vi "HEWH Adjust Temp.vi"(0 "Core HEWH Data Input":T12={"Scan Rate Adjust"=0.0, "Draw Count"=0, "Test Patten Setup"={"Total Gallons Schedule"=[], "PRAT/RLT Sequence"=[{"Sequence #"=1.0, "Cycles"=35, "Mode Setting"="", "Flow Rate (GPM)"=0.0, "Temperature (F)"=0.0, "Reset Timer"=FALSE, "Use Temp Decline Method"=FALSE, "Terminate Condition"=enum."C1-Terminate Draw @ Gallon Mark", "Condition Value #1"=0.0, "UE"=FALSE, "LE"=FALSE, "Comp"=FALSE, "Fan"=FALSE, "Test End Time (Sec)"=0.0, "Purge Until Cutout"=FALSE, "Start Conditions"=enum."Heat Source Cutout", "Condition Value #2"=0.0, "Remove Power"=FALSE, "Time"=0.0, "Check Special Cond."=enum."SC1-Do Nothing", "Condition#"=enum."C1", "Draw Flags"=enum."N/A", "Data Processing Delay (FHD 15sec, UEF 5 Sec)"=0.0, "Test Complete"=FALSE, "User Setpoint"=0.0, "Tank Setpoint"=0.0}, {"Sequence #"=2.0, "Cycles"=15, "Mode Setting"="", "Flow Rate (GPM)"=0.0, "Temperature (F)"=0.0, "Reset Timer"=FALSE, "Use Temp Decline Method"=FALSE, "Terminate Condition"=enum."C1-Terminate Draw @ Gallon Mark", "Condition Value #1"=0.0, "UE"=FALSE, "LE"=FALSE, "Comp"=FALSE, "Fan"=FALSE, "Test End Time (Sec)"=0.0, "Purge Until Cutout"=FALSE, "Start Conditions"=enum."Heat Source Cutout", "Condition Value #2"=0.0, "Remove Power"=FALSE, "Time"=0.0, "Check Special Cond."=enum."SC1-Do Nothing", "Condition#"=enum."C1", "Draw Flags"=enum."N/A", "Data Processing Delay (FHD 15sec, UEF 5 Sec)"=0.0, "Test Complete"=FALSE, "User Setpoint"=0.0, "Tank Setpoint"=0.0}, {"Sequence #"=3.0, "Cycles"=35, "Mode Setting"="", "Flow Rate (GPM)"=0.0, "Temperature (F)"=0.0, "Reset Timer"=FALSE, "Use Temp Decline Method"=FALSE, "Terminate Condition"=enum."C1-Terminate Draw @ Gallon Mark", "Condition Value #1"=0.0, "UE"=FALSE, "LE"=FALSE, "Comp"=FALSE, "Fan"=FALSE, "Test End Time (Sec)"=0.0, "Purge Until Cutout"=FALSE, "Start Conditions"=enum."Heat Source Cutout", "Condition Value #2"=0.0, "Remove Power"=FALSE, "Time"=0.0, "Check Special Cond."=enum."SC1-Do Nothing", "Condition#"=enum."C1", "Draw Flags"=enum."N/A", "Data Processing Delay (FHD 15sec, UEF 5 Sec)"=0.0, "Test Complete"=FALSE, "User Setpoint"=0.0, "Tank Setpoint"=0.0}, {"Sequence #"=4.0, "Cycles"=15, "Mode Setting"="", "Flow Rate (GPM)"=0.0, "Temperature (F)"=0.0, "Reset Timer"=FALSE, "Use Temp Decline Method"=FALSE, "Terminate Condition"=enum."C1-Terminate Draw @ Gallon Mark", "Condition Value #1"=0.0, "UE"=FALSE, "LE"=FALSE, "Comp"=FALSE, "Fan"=FALSE, "Test End Time (Sec)"=0.0, "Purge Until Cutout"=FALSE, "Start Conditions"=enum."Heat Source Cutout", "Condition Value #2"=0.0, "Remove Power"=FALSE, "Time"=0.0, "Check Special Cond."=enum."SC1-Do Nothing", "Condition#"=enum."C1", "Draw Flags"=enum."N/A", "Data Processing Delay (FHD 15sec, UEF 5 Sec)"=0.0, "Test Complete"=FALSE, "User Setpoint"=0.0, "Tank Setpoint"=0.0}, {"Sequence #"=5.0, "Cycles"=35, "Mode Setting"="", "Flow Rate (GPM)"=0.0, "Temperature (F)"=0.0, "Reset Timer"=FALSE, "Use Temp Decline Method"=FALSE, "Terminate Condition"=enum."C1-Terminate Draw @ Gallon Mark", "Condition Value #1"=0.0, "UE"=FALSE, "LE"=FALSE, "Comp"=FALSE, "Fan"=FALSE, "Test End Time (Sec)"=0.0, "Purge Until Cutout"=FALSE, "Start Conditions"=enum."Heat Source Cutout", "Condition Value #2"=0.0, "Remove Power"=FALSE, "Time"=0.0, "Check Special Cond."=enum."SC1-Do Nothing", "Condition#"=enum."C1", "Draw Flags"=enum."N/A", "Data Processing Delay (FHD 15sec, UEF 5 Sec)"=0.0, "Test Complete"=FALSE, "User Setpoint"=0.0, "Tank Setpoint"=0.0}, {"Sequence #"=6.0, "Cycles"=15, "Mode Setting"="", "Flow Rate (GPM)"=0.0, "Temperature (F)"=0.0, "Reset Timer"=FALSE, "Use Temp Decline Method"=FALSE, "Terminate Condition"=enum."C1-Terminate Draw @ Gallon Mark", "Condition Value #1"=0.0, "UE"=FALSE, "LE"=FALSE, "Comp"=FALSE, "Fan"=FALSE, "Test End Time (Sec)"=0.0, "Purge Until Cutout"=FALSE, "Start Conditions"=enum."Heat Source Cutout", "Condition Value #2"=0.0, "Remove Power"=FALSE, "Time"=0.0, "Check Special Cond."=enum."SC1-Do Nothing", "Condition#"=enum."C1", "Draw Flags"=enum."N/A", "Data Processing Delay (FHD 15sec, UEF 5 Sec)"=0.0, "Test Complete"=FALSE, "User Setpoint"=0.0, "Tank Setpoint"=0.0}, {"Sequence #"=7.0, "Cycles"=35, "Mode Setting"="", "Flow Rate (GPM)"=0.0, "Temperature (F)"=0.0, "Reset Timer"=FALSE, "Use Temp Decline Method"=FALSE, "Terminate Condition"=enum."C1-Terminate Draw @ Gallon Mark", "Condition Value #1"=0.0, "UE"=FALSE, "LE"=FALSE, "Comp"=FALSE, "Fan"=FALSE, "Test End Time (Sec)"=0.0, "Purge Until Cutout"=FALSE, "Start Conditions"=enum."Heat Source Cutout", "Condition Value #2"=0.0, "Remove Power"=FALSE, "Time"=0.0, "Check Special Cond."=enum."SC1-Do Nothing", "Condition#"=enum."C1", "Draw Flags"=enum."N/A", "Data Processing Delay (FHD 15sec, UEF 5 Sec)"=0.0, "Test Complete"=FALSE, "User Setpoint"=0.0, "Tank Setpoint"=0.0}, {"Sequence #"=8.0, "Cycles"=15, "Mode Setting"="", "Flow Rate (GPM)"=0.0, "Temperature (F)"=0.0, "Reset Timer"=FALSE, "Use Temp Decline Method"=FALSE, "Terminate Condition"=enum."C1-Terminate Draw @ Gallon Mark", "Condition Value #1"=0.0, "UE"=FALSE, "LE"=FALSE, "Comp"=FALSE, "Fan"=FALSE, "Test End Time (Sec)"=0.0, "Purge Until Cutout"=FALSE, "Start Conditions"=enum."Heat Source Cutout", "Condition Value #2"=0.0, "Remove Power"=FALSE, "Time"=0.0, "Check Special Cond."=enum."SC1-Do Nothing", "Condition#"=enum."C1", "Draw Flags"=enum."N/A", "Data Processing Delay (FHD 15sec, UEF 5 Sec)"=0.0, "Test Complete"=FALSE, "User Setpoint"=0.0, "Tank Setpoint"=0.0}], "Current Sequence Index"=0}, "HEWH Specific DAQ"={"HEWH Data"={"HEWH Standard"={"Voltage (Volts)"=0.0, "Current (Amps)"=0.0, "Power (Watts)"=0.0, "WattHours (Wh)"=0.0, "TC Tree (AVG)"=0.0, "Flow Rate (GPM)"=0.0, "Gallons (Gal)"=0.0, "RTD Out (Deg F)"=0.0, "RTD In (Deg F)"=0.0, "RTD Amb (Deg F)"=0.0, "TC Down"=0.0, "UE Event Lead"=0, "LE Event Lead"=0, "TC 8"=0.0, "TC 9"=0.0, "TC 10"=0.0, "TC Tree Array (1-6)"=[], "TC 7"=0.0, "PSI 1"=0.0, "PSI 2"=0.0, "PSI 3"=0.0, "PSI 4"=0.0, "Gas BTU"=0.0, "Gas BTU/hr"=0.0}, "PRAT"={"Power (Watts) A"=4192.0, "Power (Watts) B"=4192.0, "Power (Watts) C"=4192.0, "Power (Watts) D"=4192.0, "TC1"=0.0, "TC2"=0.0, "TC3"=0.0, "TC4"=0.0, "WattHours (Wh) A"=4192.0, "WattHours (Wh) B"=4192.0, "WattHours (Wh) C"=4192.0, "WattHours (Wh) D"=4192.0, "Ambient"=0.0, "Extra Temp"=0.0}, "Additional Power Data"={"Vthd"=236.2, "Frequency (Hz)"=236.2, "Apparent Power (VA)"=236.2, "Power Factor"=236.2, "Current Crest Factor"=236.2, "Voltage Crest Factor"=236.2, "Integration Time (sec)"=236.2}}, "Flow Valve % Open"=0.0, "Power State"={"UE"=FALSE, "LE"=FALSE, "COMP"=FALSE, "FANS"=FALSE}, "Power Analyzer"=enum."APLUS", "Flow Valve uA Output"=0, "Gallons Start (Gal)"=0.0, "PI Output"=0.0}, "Test Output Data"={"PreDraw Data Table"=[], "Data Table"=[], "MW100 TC Headers"=[]}, "Calc and Calibration"={"Mean SD Var Max Min Array"=[], "Draw Statistics (DBL)"=[], "Calibration Coefficients DBL"=[], "Start Gallons"=0.0, "Starting Temp Decline"=0.0, "K-Factor (Temperature)"=0.0, "All Draw Stats"=[], "RTD Terminate Value"=0.0, "K-Factor (Flow)"=0.0, "Intellifaucet Type"="", "Thermal Stabil Array"=[], "Gas Thermal Stabil Complete"=FALSE, "Therm Reset Cmpt 1"=FALSE, "Therm Reset Cmpt 2"=FALSE, "Last Flow Rate (Therm)"=0.0, "State"=enum."State 1", "Gas Thermal Time"=0.0, "Target Rate (Thermal)"=0.0, "Thermal - Final"=[], "State5 Gal Water"=0.0, "State 5 Gal Gas"=0.0, "Intellif Open < 1"=0.0, "Intellif Open < 1.7"=0.0, "Intellif Open < 2.2"=0.0, "Intellif Open > 2.2"=0.0, "End of Draw\nComparison"=[]}, "Current Draw Time"=0.0, "LV Program"=enum."HEWH", "Station ID"=enum."A", "Current Cond"=enum."N/A", "Test Complete"=FALSE, "ANSI Rate"={"Array 1"=[], "Array 3"=[], "Array 2"=[], "Start ANSI"=FALSE, "ANSI Start Time"=0.0, "Restart ANSI"=FALSE, "15 Min ANSI Avg (BTU/hr)"=0.0, "20 Min ANSI Avg (BTU/hr)"=0.0, "25 Min ANSI Avg (BTU/hr)"=0.0, "Absolute Pressure"=0.0, "Gas Temperature"=0.0, "Volumetric Flow Rate"=0.0, "Mass Flow Rate"=0.0, "Array 4"=[], "Array 5"=[], "Gas Rate"=0.0, "15 Min Pres Avg (PSIA)"=0.0, "20 Min Pres Avg (PSIA)"=0.0, "25 Min Pres Avg (PSIA)"=0.0, "15 Min Temp Avg (°F) "=0.0, "20 Min Temp Avg (°F)"=0.0, "25 Min Temp Avg (°F)"=0.0, "15 Min Uncorrected Avg (CFH)"=0.0, "20 Min Uncorrected Avg (CFH)"=0.0, "25 Min Uncorrected Avg (CFH)"=0.0, "15 Min Corrected Avg (SCFH)"=0.0, "20 Min Corrected Avg (SCFH)"=0.0, "25 Min Corrected Avg (SCFH)"=0.0, "15 Min Complete"=FALSE, "20 Min Complete"=FALSE, "25 Min Complete"=FALSE, "Heating Value (BTU/ft³)"=0.0, "CO CO2 15 Min"=[], "CO CO2 20 Min"=[], "CO CO2 25 Min"=[], "CO CO2 Real Time"=[]}, "Module 4 Relay Status"={"INTELLIFAUCET TEMP(T)/FLOW(F) (CH 041)"=FALSE, "INTELLIFAUCET READY (CH 042)"=FALSE, "INTELLIFAUCET START (CH 043)"=FALSE, "INTELLIFAUCET STOP (CH 044)"=FALSE, "MAIN POWER RELAY (CH 047)"=FALSE, "NOT USED (CH 045)"=FALSE, "NOT USED (CH 046)"=FALSE, "PURGE VALVE RELAY (CH 048)"=FALSE, "OUTLET VALVE RELAY (CH 049)"=FALSE, "INLET VALVE RELAY (CH 050)"=FALSE, "Intellifaucet (% Open)"=0.0, "Proportioning Valve (%Open)"=0.0, "Intellifaucet Temp Setpoint (F)"=0.0}, "Inficon Data Output"={"Gross Heating Value, Vol (Real, Dry)"=1067.4462890625, "Nitrogen Component Normalized Mole % (Dry)"=0.0, "Methane Component Normalized Mole % (Dry)"=92.87550354003906, "Carbon Dioxide Component Normalized Mole % (Dry)"=0.1941000074148178, "Ethane Component Normalized Mole % (Dry)"=6.454999923706055, "Propane Component Normalized Mole % (Dry)"=0.3865000009536743, "i-Pentane Component Normalized Mole % (Dry)"=0.007799999788403511, "i-Butane Component Normalized Mole % (Dry)"=0.03880000114440918, "n-Butane Component Normalized Mole % (Dry)"=0.03819999843835831, "n-Pentane Component Normalized Mole % (Dry)"=0.004100000020116568, "Hexane Component Normalized Mole % (Dry)"=0.0, "Heptane Component Normalized Mole % (Dry)"=0.0, "Gross Wobbe Index, Real(Dry)"=1385.8905029296875, "Relative Density, Real(Dry)"=0.5932452082633972, "Propylene Component Normalized Mole % (Dry)"=0.0, "C4 Olefins Component Normalized Mole % (Dry)"=0.0, "Water Component Normalized Mole % (Dry)"=0.0, "Gross Heating Value, Vol (Real, Sat)"=0.0}, "Gas Measurements"={"Gas Measurment Data -Alicat"={"Absolute Pressure"=0.0, "Gauge/Diff. Pressure"=0.0, "Barometric Pressure"=0.0, "Temperature"=0.0, "Volumetric Flow"=0.0, "Mass Flow"=0.0, "Setpoint"=0.0, "Valve Drive"=0.0, "Totalizer"=0.0, "[hr]"=0.0, "[min]"=0.0, "[sec]"=0.0, "Totalizer Average Flow"=0.0, "Totalizer Peak Flow"=0.0, "Gas selected"=""}, "Gas Measurment Data - Ritter"={"Gas Flow Rate (L/hr)-Uncorrected"=0.0, "Totalized Flow (L)--Uncorrected"=0.0, "Gas Flow Rate (cuft/hr)-Uncorrected"=0.0, "Totalized Flow (cuft)-Uncorrected"=0.0, "Gas Temperature (F)"=0.0, "Gas Pressure (in WC)"=0.0, "Heise Barometric Pressure (inHG)"=0.0, "STP Correction Factor"=0.0, "Temp Correction Factor"=0.0, "Pressure Correction Factor"=0.0, "Water Vapor Pressure"=0.0, "Gas Flow Rate (cuft/hr)-Corrected"=0.0, "Totalized Flow (cuft)-Corrected"=0.0}}} {"Test Patten Setup"."PRAT/RLT Sequence"."Time" format="%<%H:%M:%S>t"; "Test Patten Setup"."Total Gallons Schedule" format="%.2f"}, 1 "Test Fixture Hardware":T1={"Power "={"Yokogawa"={"WT210"={"Sample Rate (1: 0.25s)"=1, "A Range (12: 20A)"=11, "V Range (6: 600V)"=4, "Power VISA Yokogawa WT210"="WT210"}, "WT500"={"Power VISA Yokogawa WT500"="", "V Range (8: 1000V)"=6, "I Range (7: 40A)"=7, "Update Rate (3: 500ms)"=2}, "WT310_2"={"Sample Rate (1: 0.25s)"=1, "A Range (12: 20A)"=11, "V Range (6: 600V)"=4, "Power VISA Yokogawa WT310_2"="WT310_2"}, "WT310_3"={"Sample Rate (1: 0.25s)"=1, "A Range (12: 20A)"=11, "V Range (6: 600V)"=4, "Power VISA Yokogawa WT310_3"="WT310_3"}}, "Aplus"={"Aplus IP Address"="192.168.1.101", "Remote Port"=502, "Instrument"="APLUS", "Instr Driver Revision"="1.03.0053"}, "Power Limits"={"Crest Factor"={"Upper Limit"=1.49, "Lower Limit"=1.34}, "Harmonic Content"={"Uthd"=2.0}, "Voltage"={"% Error"=2.0}, "Stability"={"<1 Watt "={"Wattage"=1.0, "Slope (mW/H)"=10.0}, ">1 Watt"={"1%Power/Hour"=1.0}}}, "Nominal Voltage"=120, "Time Limit (s)"=10800.0, "Power Variation Limit (%)"=50.0, "Power Supply"={"Chroma 61605"="CHROMA", "Use Chroma?"=FALSE}}, "Weight Scale"={"Com Options"={"IND560Scale VISA"="IND560", "IP Address"="", "Remote Port"=502, "Setra Scale VISA"="SETRA", "GSE 350"="GSE350"}, "Select Scale"=""}, "Flow Rates"={"Laurel Cold IP Address"="", "Laurel Hot IP Address"="", "Hot Water Laurel VISA"="LaurelMeter_Hot", "Cold Water Laurel VISA"="LaurelMeter_Cold", "Remote Port"=0, "Laurel Communication Type"="", "Meters To Collect (Hot Cold)"="", "HOT Laurel Reference"=refnum, "COLD Laurel Reference"=refnum, "Modbus Hot Ref"=refnum}, "Analog Data"={"Agilent"={"Agilent 34972_1"="34972A_1", "Agilent 34972_2"="34972A_2", "Agilent 34972_3"="34972A_3", "Agilent 34972_4"="34972A_3", "Agilent 34972_5"="34972A_3", "Agilent 34972_6"="34972A_3", "Agilent Gain"=0.0, "TC Type (K,J,T)"="", "Instrument IDN?"="", "TC Channels-List"="", "Analog Channels-List"="", "Agilent Cluster Array"=[], "TC Channels-List 2"="", "Analog Channels-List 2"=""}, "Yokogawa"={"MW100"="MW100", "Intellifaucet"=FALSE}, "Select Analog"="", "TC Coefficients"={"TC Coefficients 1"=[], "TC Coefficients 2"=[], "TC Coefficients 3"=[], "TC Coefficients 4"=[], "TC Coefficients 5"=[], "TC Coefficients 6"=[], "TC Coefficients 7"=[]}, "NI Tasks (Dryer DOE)"=["TC Temps-Module 1", "TC Temps-Module 2", "TC Temps-Module 3", "TC Temps-Module 4", "TC Temps-Module 5", "Gas and Temp-Module 6", "AC_DC Events-Module 7"], "Laurel Analog"={"Laurel IP (Water Temp)"="", "Laurel IP (Pressure)"=""}}, "ITHX-Temp Humidity"={"IP Address 1"="", "Remote Port"=0, "IP Address 2"="", "IP Address 3"=""}, "Gas Meter"={"Gas Meter 1"="COM3", "Gas Meter 2"="COM4", "Gas Meter 3"="COM5", "Gas Meter 4"="COM6", "Gas Meter 5"="COM7", "Gas Meter 6"="COM8", "Data Frame Format"={"Absolute Pressure"=FALSE, "Gauge/Diff. Pressure"=FALSE, "Barometric Pressure"=FALSE, "Temperature"=FALSE, "Volumetric"=FALSE, "Mass"=FALSE, "Setpoint"=FALSE, "Valve Drive"=FALSE, "Totalizer"=FALSE, "Totalizer Timer"=FALSE, "Totalizer Average Flow"=FALSE, "Totalizer Peak Flow"=FALSE, "Gas Selected"=FALSE, "Tot. Timer Format"=0}, "Measurement Units"={"Software Rev"="", "Model Number"="", "Manufacturer Info"="", "Software Sub-Rev"="", "Board Rev"="", "Units of Measure Input"={"Abs. Pressure"="", "Gauge/Diff. Press."="", "Barometric Press."="", "Temperature"="", "Volume"="", "Mass"="", "Setpoint"="", "Valve Drive"="", "Totalizer"="", "Tot. Timer"="", "Tot. Avg. Flow"="", "Tot. Peak Flow"=""}}, "Ritter Gas Meter 1"="COM8"}, "Barometric Pressure"={"HEISE 901A"="HEISE", "Use Barometer?"=FALSE}, "Gas Analysis"={"Ultramat 23 VISA"="ULTRAMAT"}, "Inficon Micro GC"={"Propane IP Address"="192.168.1.33", "Natural Gas  IP Address"="192.168.1.32", "Remote Port"=502, "Natural Modbus"=refnum, "Propane Modbus"=refnum}} {"Power"."Yokogawa"."WT310_3"."V Range (6: 600V)" items=["Auto", "15V", "30V", "60V", "150V", "300V", "600V"]; "Power"."Yokogawa"."WT310_3"."A Range (12: 20A)" items=["Auto", "5mA", "10mA", "20mA", "50mA", "100mA", "200mA", "0.5A", "1A", "2A", "5A", "10A", "20A", "50mV", "100mV", "200mV", "2.5V", "5V", "10V"]; "Power"."Yokogawa"."WT310_3"."Sample Rate (1: 0.25s)" items=["0.1s", "0.25s", "0.5s", "1s", "2s", "5s"]; "Power"."Yokogawa"."WT310_2"."V Range (6: 600V)" items=["Auto", "15V", "30V", "60V", "150V", "300V", "600V"]; "Power"."Yokogawa"."WT310_2"."A Range (12: 20A)" items=["Auto", "5mA", "10mA", "20mA", "50mA", "100mA", "200mA", "0.5A", "1A", "2A", "5A", "10A", "20A", "50mV", "100mV", "200mV", "2.5V", "5V", "10V"]; "Power"."Yokogawa"."WT310_2"."Sample Rate (1: 0.25s)" items=["0.1s", "0.25s", "0.5s", "1s", "2s", "5s"]; "Power"."Yokogawa"."WT500"."Update Rate (3: 500ms)" items=["-", "100ms", "200ms", "500ms", "1s", "2s", "5s"]; "Power"."Yokogawa"."WT500"."I Range (7: 40A)" items=["AUTO", "500 mA", "1 A", "2 A", "5 A", "10 A", "20 A", "40 A", "S-AUTO", "50 mV", "100 mV", "200 mV", "500 mV", "1 V", "2 V", "5 V", "10 V", "250 mA", "500 mA", "1 A", "2.5 A", "5 A", "10 A", "20 A", "25 mV", "50 mV", "100 mV", "250 mV", "500 mV", "1 V", "2.5 V", "5 V"]; "Power"."Yokogawa"."WT500"."V Range (8: 1000V)" items=["AUTO", "15", "30", "60", "100", "150", "300", "600", "1000", "7.5", "15", "30", "50", "75", "150", "300", "500"]; "Power"."Yokogawa"."WT210"."V Range (6: 600V)" items=["Auto", "15V", "30V", "60V", "150V", "300V", "600V"]; "Power"."Yokogawa"."WT210"."A Range (12: 20A)" items=["Auto", "5mA", "10mA", "20mA", "50mA", "100mA", "200mA", "0.5A", "1A", "2A", "5A", "10A", "20A", "50mV", "100mV", "200mV", "2.5V", "5V", "10V"]; "Power"."Yokogawa"."WT210"."Sample Rate (1: 0.25s)" items=["0.1s", "0.25s", "0.5s", "1s", "2s", "5s"]}, 4 "MW100 Sema":T11, 5 "error in (no error)":errorcluster, 7 "Debug":bool, 9 "Temperature":T32 format="%.2f", 13 "Adjust Temp":bool) -> (14 "Core HEWH Data Output":T12={"Scan Rate Adjust"=0.0, "Draw Count"=0, "Test Patten Setup"={"Total Gallons Schedule"=[], "PRAT/RLT Sequence"=[{"Sequence #"=1.0, "Cycles"=35, "Mode Setting"="", "Flow Rate (GPM)"=0.0, "Temperature (F)"=0.0, "Reset Timer"=FALSE, "Use Temp Decline Method"=FALSE, "Terminate Condition"=enum."C1-Terminate Draw @ Gallon Mark", "Condition Value #1"=0.0, "UE"=FALSE, "LE"=FALSE, "Comp"=FALSE, "Fan"=FALSE, "Test End Time (Sec)"=0.0, "Purge Until Cutout"=FALSE, "Start Conditions"=enum."Heat Source Cutout", "Condition Value #2"=0.0, "Remove Power"=FALSE, "Time"=0.0, "Check Special Cond."=enum."SC1-Do Nothing", "Condition#"=enum."C1", "Draw Flags"=enum."N/A", "Data Processing Delay (FHD 15sec, UEF 5 Sec)"=0.0, "Test Complete"=FALSE, "User Setpoint"=0.0, "Tank Setpoint"=0.0}, {"Sequence #"=2.0, "Cycles"=15, "Mode Setting"="", "Flow Rate (GPM)"=0.0, "Temperature (F)"=0.0, "Reset Timer"=FALSE, "Use Temp Decline Method"=FALSE, "Terminate Condition"=enum."C1-Terminate Draw @ Gallon Mark", "Condition Value #1"=0.0, "UE"=FALSE, "LE"=FALSE, "Comp"=FALSE, "Fan"=FALSE, "Test End Time (Sec)"=0.0, "Purge Until Cutout"=FALSE, "Start Conditions"=enum."Heat Source Cutout", "Condition Value #2"=0.0, "Remove Power"=FALSE, "Time"=0.0, "Check Special Cond."=enum."SC1-Do Nothing", "Condition#"=enum."C1", "Draw Flags"=enum."N/A", "Data Processing Delay (FHD 15sec, UEF 5 Sec)"=0.0, "Test Complete"=FALSE, "User Setpoint"=0.0, "Tank Setpoint"=0.0}, {"Sequence #"=3.0, "Cycles"=35, "Mode Setting"="", "Flow Rate (GPM)"=0.0, "Temperature (F)"=0.0, "Reset Timer"=FALSE, "Use Temp Decline Method"=FALSE, "Terminate Condition"=enum."C1-Terminate Draw @ Gallon Mark", "Condition Value #1"=0.0, "UE"=FALSE, "LE"=FALSE, "Comp"=FALSE, "Fan"=FALSE, "Test End Time (Sec)"=0.0, "Purge Until Cutout"=FALSE, "Start Conditions"=enum."Heat Source Cutout", "Condition Value #2"=0.0, "Remove Power"=FALSE, "Time"=0.0, "Check Special Cond."=enum."SC1-Do Nothing", "Condition#"=enum."C1", "Draw Flags"=enum."N/A", "Data Processing Delay (FHD 15sec, UEF 5 Sec)"=0.0, "Test Complete"=FALSE, "User Setpoint"=0.0, "Tank Setpoint"=0.0}, {"Sequence #"=4.0, "Cycles"=15, "Mode Setting"="", "Flow Rate (GPM)"=0.0, "Temperature (F)"=0.0, "Reset Timer"=FALSE, "Use Temp Decline Method"=FALSE, "Terminate Condition"=enum."C1-Terminate Draw @ Gallon Mark", "Condition Value #1"=0.0, "UE"=FALSE, "LE"=FALSE, "Comp"=FALSE, "Fan"=FALSE, "Test End Time (Sec)"=0.0, "Purge Until Cutout"=FALSE, "Start Conditions"=enum."Heat Source Cutout", "Condition Value #2"=0.0, "Remove Power"=FALSE, "Time"=0.0, "Check Special Cond."=enum."SC1-Do Nothing", "Condition#"=enum."C1", "Draw Flags"=enum."N/A", "Data Processing Delay (FHD 15sec, UEF 5 Sec)"=0.0, "Test Complete"=FALSE, "User Setpoint"=0.0, "Tank Setpoint"=0.0}, {"Sequence #"=5.0, "Cycles"=35, "Mode Setting"="", "Flow Rate (GPM)"=0.0, "Temperature (F)"=0.0, "Reset Timer"=FALSE, "Use Temp Decline Method"=FALSE, "Terminate Condition"=enum."C1-Terminate Draw @ Gallon Mark", "Condition Value #1"=0.0, "UE"=FALSE, "LE"=FALSE, "Comp"=FALSE, "Fan"=FALSE, "Test End Time (Sec)"=0.0, "Purge Until Cutout"=FALSE, "Start Conditions"=enum."Heat Source Cutout", "Condition Value #2"=0.0, "Remove Power"=FALSE, "Time"=0.0, "Check Special Cond."=enum."SC1-Do Nothing", "Condition#"=enum."C1", "Draw Flags"=enum."N/A", "Data Processing Delay (FHD 15sec, UEF 5 Sec)"=0.0, "Test Complete"=FALSE, "User Setpoint"=0.0, "Tank Setpoint"=0.0}, {"Sequence #"=6.0, "Cycles"=15, "Mode Setting"="", "Flow Rate (GPM)"=0.0, "Temperature (F)"=0.0, "Reset Timer"=FALSE, "Use Temp Decline Method"=FALSE, "Terminate Condition"=enum."C1-Terminate Draw @ Gallon Mark", "Condition Value #1"=0.0, "UE"=FALSE, "LE"=FALSE, "Comp"=FALSE, "Fan"=FALSE, "Test End Time (Sec)"=0.0, "Purge Until Cutout"=FALSE, "Start Conditions"=enum."Heat Source Cutout", "Condition Value #2"=0.0, "Remove Power"=FALSE, "Time"=0.0, "Check Special Cond."=enum."SC1-Do Nothing", "Condition#"=enum."C1", "Draw Flags"=enum."N/A", "Data Processing Delay (FHD 15sec, UEF 5 Sec)"=0.0, "Test Complete"=FALSE, "User Setpoint"=0.0, "Tank Setpoint"=0.0}, {"Sequence #"=7.0, "Cycles"=35, "Mode Setting"="", "Flow Rate (GPM)"=0.0, "Temperature (F)"=0.0, "Reset Timer"=FALSE, "Use Temp Decline Method"=FALSE, "Terminate Condition"=enum."C1-Terminate Draw @ Gallon Mark", "Condition Value #1"=0.0, "UE"=FALSE, "LE"=FALSE, "Comp"=FALSE, "Fan"=FALSE, "Test End Time (Sec)"=0.0, "Purge Until Cutout"=FALSE, "Start Conditions"=enum."Heat Source Cutout", "Condition Value #2"=0.0, "Remove Power"=FALSE, "Time"=0.0, "Check Special Cond."=enum."SC1-Do Nothing", "Condition#"=enum."C1", "Draw Flags"=enum."N/A", "Data Processing Delay (FHD 15sec, UEF 5 Sec)"=0.0, "Test Complete"=FALSE, "User Setpoint"=0.0, "Tank Setpoint"=0.0}, {"Sequence #"=8.0, "Cycles"=15, "Mode Setting"="", "Flow Rate (GPM)"=0.0, "Temperature (F)"=0.0, "Reset Timer"=FALSE, "Use Temp Decline Method"=FALSE, "Terminate Condition"=enum."C1-Terminate Draw @ Gallon Mark", "Condition Value #1"=0.0, "UE"=FALSE, "LE"=FALSE, "Comp"=FALSE, "Fan"=FALSE, "Test End Time (Sec)"=0.0, "Purge Until Cutout"=FALSE, "Start Conditions"=enum."Heat Source Cutout", "Condition Value #2"=0.0, "Remove Power"=FALSE, "Time"=0.0, "Check Special Cond."=enum."SC1-Do Nothing", "Condition#"=enum."C1", "Draw Flags"=enum."N/A", "Data Processing Delay (FHD 15sec, UEF 5 Sec)"=0.0, "Test Complete"=FALSE, "User Setpoint"=0.0, "Tank Setpoint"=0.0}], "Current Sequence Index"=0}, "HEWH Specific DAQ"={"HEWH Data"={"HEWH Standard"={"Voltage (Volts)"=0.0, "Current (Amps)"=0.0, "Power (Watts)"=0.0, "WattHours (Wh)"=0.0, "TC Tree (AVG)"=0.0, "Flow Rate (GPM)"=0.0, "Gallons (Gal)"=0.0, "RTD Out (Deg F)"=0.0, "RTD In (Deg F)"=0.0, "RTD Amb (Deg F)"=0.0, "TC Down"=0.0, "UE Event Lead"=0, "LE Event Lead"=0, "TC 8"=0.0, "TC 9"=0.0, "TC 10"=0.0, "TC Tree Array (1-6)"=[], "TC 7"=0.0, "PSI 1"=0.0, "PSI 2"=0.0, "PSI 3"=0.0, "PSI 4"=0.0, "Gas BTU"=0.0, "Gas BTU/hr"=0.0}, "PRAT"={"Power (Watts) A"=4192.0, "Power (Watts) B"=4192.0, "Power (Watts) C"=4192.0, "Power (Watts) D"=4192.0, "TC1"=0.0, "TC2"=0.0, "TC3"=0.0, "TC4"=0.0, "WattHours (Wh) A"=4192.0, "WattHours (Wh) B"=4192.0, "WattHours (Wh) C"=4192.0, "WattHours (Wh) D"=4192.0, "Ambient"=0.0, "Extra Temp"=0.0}, "Additional Power Data"={"Vthd"=236.2, "Frequency (Hz)"=236.2, "Apparent Power (VA)"=236.2, "Power Factor"=236.2, "Current Crest Factor"=236.2, "Voltage Crest Factor"=236.2, "Integration Time (sec)"=236.2}}, "Flow Valve % Open"=0.0, "Power State"={"UE"=FALSE, "LE"=FALSE, "COMP"=FALSE, "FANS"=FALSE}, "Power Analyzer"=enum."APLUS", "Flow Valve uA Output"=0, "Gallons Start (Gal)"=0.0, "PI Output"=0.0}, "Test Output Data"={"PreDraw Data Table"=[], "Data Table"=[], "MW100 TC Headers"=[]}, "Calc and Calibration"={"Mean SD Var Max Min Array"=[], "Draw Statistics (DBL)"=[], "Calibration Coefficients DBL"=[], "Start Gallons"=0.0, "Starting Temp Decline"=0.0, "K-Factor (Temperature)"=0.0, "All Draw Stats"=[], "RTD Terminate Value"=0.0, "K-Factor (Flow)"=0.0, "Intellifaucet Type"="", "Thermal Stabil Array"=[], "Gas Thermal Stabil Complete"=FALSE, "Therm Reset Cmpt 1"=FALSE, "Therm Reset Cmpt 2"=FALSE, "Last Flow Rate (Therm)"=0.0, "State"=enum."State 1", "Gas Thermal Time"=0.0, "Target Rate (Thermal)"=0.0, "Thermal - Final"=[], "State5 Gal Water"=0.0, "State 5 Gal Gas"=0.0, "Intellif Open < 1"=0.0, "Intellif Open < 1.7"=0.0, "Intellif Open < 2.2"=0.0, "Intellif Open > 2.2"=0.0, "End of Draw\nComparison"=[]}, "Current Draw Time"=0.0, "LV Program"=enum."HEWH", "Station ID"=enum."A", "Current Cond"=enum."N/A", "Test Complete"=FALSE, "ANSI Rate"={"Array 1"=[], "Array 3"=[], "Array 2"=[], "Start ANSI"=FALSE, "ANSI Start Time"=0.0, "Restart ANSI"=FALSE, "15 Min ANSI Avg (BTU/hr)"=0.0, "20 Min ANSI Avg (BTU/hr)"=0.0, "25 Min ANSI Avg (BTU/hr)"=0.0, "Absolute Pressure"=0.0, "Gas Temperature"=0.0, "Volumetric Flow Rate"=0.0, "Mass Flow Rate"=0.0, "Array 4"=[], "Array 5"=[], "Gas Rate"=0.0, "15 Min Pres Avg (PSIA)"=0.0, "20 Min Pres Avg (PSIA)"=0.0, "25 Min Pres Avg (PSIA)"=0.0, "15 Min Temp Avg (°F) "=0.0, "20 Min Temp Avg (°F)"=0.0, "25 Min Temp Avg (°F)"=0.0, "15 Min Uncorrected Avg (CFH)"=0.0, "20 Min Uncorrected Avg (CFH)"=0.0, "25 Min Uncorrected Avg (CFH)"=0.0, "15 Min Corrected Avg (SCFH)"=0.0, "20 Min Corrected Avg (SCFH)"=0.0, "25 Min Corrected Avg (SCFH)"=0.0, "15 Min Complete"=FALSE, "20 Min Complete"=FALSE, "25 Min Complete"=FALSE, "Heating Value (BTU/ft³)"=0.0, "CO CO2 15 Min"=[], "CO CO2 20 Min"=[], "CO CO2 25 Min"=[], "CO CO2 Real Time"=[]}, "Module 4 Relay Status"={"INTELLIFAUCET TEMP(T)/FLOW(F) (CH 041)"=FALSE, "INTELLIFAUCET READY (CH 042)"=FALSE, "INTELLIFAUCET START (CH 043)"=FALSE, "INTELLIFAUCET STOP (CH 044)"=FALSE, "MAIN POWER RELAY (CH 047)"=FALSE, "NOT USED (CH 045)"=FALSE, "NOT USED (CH 046)"=FALSE, "PURGE VALVE RELAY (CH 048)"=FALSE, "OUTLET VALVE RELAY (CH 049)"=FALSE, "INLET VALVE RELAY (CH 050)"=FALSE, "Intellifaucet (% Open)"=0.0, "Proportioning Valve (%Open)"=0.0, "Intellifaucet Temp Setpoint (F)"=0.0}, "Inficon Data Output"={"Gross Heating Value, Vol (Real, Dry)"=1067.4462890625, "Nitrogen Component Normalized Mole % (Dry)"=0.0, "Methane Component Normalized Mole % (Dry)"=92.87550354003906, "Carbon Dioxide Component Normalized Mole % (Dry)"=0.1941000074148178, "Ethane Component Normalized Mole % (Dry)"=6.454999923706055, "Propane Component Normalized Mole % (Dry)"=0.3865000009536743, "i-Pentane Component Normalized Mole % (Dry)"=0.007799999788403511, "i-Butane Component Normalized Mole % (Dry)"=0.03880000114440918, "n-Butane Component Normalized Mole % (Dry)"=0.03819999843835831, "n-Pentane Component Normalized Mole % (Dry)"=0.004100000020116568, "Hexane Component Normalized Mole % (Dry)"=0.0, "Heptane Component Normalized Mole % (Dry)"=0.0, "Gross Wobbe Index, Real(Dry)"=1385.8905029296875, "Relative Density, Real(Dry)"=0.5932452082633972, "Propylene Component Normalized Mole % (Dry)"=0.0, "C4 Olefins Component Normalized Mole % (Dry)"=0.0, "Water Component Normalized Mole % (Dry)"=0.0, "Gross Heating Value, Vol (Real, Sat)"=0.0}, "Gas Measurements"={"Gas Measurment Data -Alicat"={"Absolute Pressure"=0.0, "Gauge/Diff. Pressure"=0.0, "Barometric Pressure"=0.0, "Temperature"=0.0, "Volumetric Flow"=0.0, "Mass Flow"=0.0, "Setpoint"=0.0, "Valve Drive"=0.0, "Totalizer"=0.0, "[hr]"=0.0, "[min]"=0.0, "[sec]"=0.0, "Totalizer Average Flow"=0.0, "Totalizer Peak Flow"=0.0, "Gas selected"=""}, "Gas Measurment Data - Ritter"={"Gas Flow Rate (L/hr)-Uncorrected"=0.0, "Totalized Flow (L)--Uncorrected"=0.0, "Gas Flow Rate (cuft/hr)-Uncorrected"=0.0, "Totalized Flow (cuft)-Uncorrected"=0.0, "Gas Temperature (F)"=0.0, "Gas Pressure (in WC)"=0.0, "Heise Barometric Pressure (inHG)"=0.0, "STP Correction Factor"=0.0, "Temp Correction Factor"=0.0, "Pressure Correction Factor"=0.0, "Water Vapor Pressure"=0.0, "Gas Flow Rate (cuft/hr)-Corrected"=0.0, "Totalized Flow (cuft)-Corrected"=0.0}}} {"Test Patten Setup"."PRAT/RLT Sequence"."Time" format="%<%H:%M:%S>t"; "Test Patten Setup"."Total Gallons Schedule" format="%.2f"}, 15 "Test Fixture Hardware Output":T1={"Power "={"Yokogawa"={"WT210"={"Sample Rate (1: 0.25s)"=1, "A Range (12: 20A)"=11, "V Range (6: 600V)"=4, "Power VISA Yokogawa WT210"="WT210"}, "WT500"={"Power VISA Yokogawa WT500"="", "V Range (8: 1000V)"=6, "I Range (7: 40A)"=7, "Update Rate (3: 500ms)"=2}, "WT310_2"={"Sample Rate (1: 0.25s)"=1, "A Range (12: 20A)"=11, "V Range (6: 600V)"=4, "Power VISA Yokogawa WT310_2"="WT310_2"}, "WT310_3"={"Sample Rate (1: 0.25s)"=1, "A Range (12: 20A)"=11, "V Range (6: 600V)"=4, "Power VISA Yokogawa WT310_3"="WT310_3"}}, "Aplus"={"Aplus IP Address"="192.168.1.101", "Remote Port"=502, "Instrument"="APLUS", "Instr Driver Revision"="1.03.0053"}, "Power Limits"={"Crest Factor"={"Upper Limit"=1.49, "Lower Limit"=1.34}, "Harmonic Content"={"Uthd"=2.0}, "Voltage"={"% Error"=2.0}, "Stability"={"<1 Watt "={"Wattage"=1.0, "Slope (mW/H)"=10.0}, ">1 Watt"={"1%Power/Hour"=1.0}}}, "Nominal Voltage"=120, "Time Limit (s)"=10800.0, "Power Variation Limit (%)"=50.0, "Power Supply"={"Chroma 61605"="CHROMA", "Use Chroma?"=FALSE}}, "Weight Scale"={"Com Options"={"IND560Scale VISA"="IND560", "IP Address"="", "Remote Port"=502, "Setra Scale VISA"="SETRA", "GSE 350"="GSE350"}, "Select Scale"=""}, "Flow Rates"={"Laurel Cold IP Address"="", "Laurel Hot IP Address"="", "Hot Water Laurel VISA"="LaurelMeter_Hot", "Cold Water Laurel VISA"="LaurelMeter_Cold", "Remote Port"=0, "Laurel Communication Type"="", "Meters To Collect (Hot Cold)"="", "HOT Laurel Reference"=refnum, "COLD Laurel Reference"=refnum, "Modbus Hot Ref"=refnum}, "Analog Data"={"Agilent"={"Agilent 34972_1"="34972A_1", "Agilent 34972_2"="34972A_2", "Agilent 34972_3"="34972A_3", "Agilent 34972_4"="34972A_3", "Agilent 34972_5"="34972A_3", "Agilent 34972_6"="34972A_3", "Agilent Gain"=0.0, "TC Type (K,J,T)"="", "Instrument IDN?"="", "TC Channels-List"="", "Analog Channels-List"="", "Agilent Cluster Array"=[], "TC Channels-List 2"="", "Analog Channels-List 2"=""}, "Yokogawa"={"MW100"="MW100", "Intellifaucet"=FALSE}, "Select Analog"="", "TC Coefficients"={"TC Coefficients 1"=[], "TC Coefficients 2"=[], "TC Coefficients 3"=[], "TC Coefficients 4"=[], "TC Coefficients 5"=[], "TC Coefficients 6"=[], "TC Coefficients 7"=[]}, "NI Tasks (Dryer DOE)"=["TC Temps-Module 1", "TC Temps-Module 2", "TC Temps-Module 3", "TC Temps-Module 4", "TC Temps-Module 5", "Gas and Temp-Module 6", "AC_DC Events-Module 7"], "Laurel Analog"={"Laurel IP (Water Temp)"="", "Laurel IP (Pressure)"=""}}, "ITHX-Temp Humidity"={"IP Address 1"="", "Remote Port"=0, "IP Address 2"="", "IP Address 3"=""}, "Gas Meter"={"Gas Meter 1"="COM3", "Gas Meter 2"="COM4", "Gas Meter 3"="COM5", "Gas Meter 4"="COM6", "Gas Meter 5"="COM7", "Gas Meter 6"="COM8", "Data Frame Format"={"Absolute Pressure"=FALSE, "Gauge/Diff. Pressure"=FALSE, "Barometric Pressure"=FALSE, "Temperature"=FALSE, "Volumetric"=FALSE, "Mass"=FALSE, "Setpoint"=FALSE, "Valve Drive"=FALSE, "Totalizer"=FALSE, "Totalizer Timer"=FALSE, "Totalizer Average Flow"=FALSE, "Totalizer Peak Flow"=FALSE, "Gas Selected"=FALSE, "Tot. Timer Format"=0}, "Measurement Units"={"Software Rev"="", "Model Number"="", "Manufacturer Info"="", "Software Sub-Rev"="", "Board Rev"="", "Units of Measure Input"={"Abs. Pressure"="", "Gauge/Diff. Press."="", "Barometric Press."="", "Temperature"="", "Volume"="", "Mass"="", "Setpoint"="", "Valve Drive"="", "Totalizer"="", "Tot. Timer"="", "Tot. Avg. Flow"="", "Tot. Peak Flow"=""}}, "Ritter Gas Meter 1"="COM8"}, "Barometric Pressure"={"HEISE 901A"="HEISE", "Use Barometer?"=FALSE}, "Gas Analysis"={"Ultramat 23 VISA"="ULTRAMAT"}, "Inficon Micro GC"={"Propane IP Address"="192.168.1.33", "Natural Gas  IP Address"="192.168.1.32", "Remote Port"=502, "Natural Modbus"=refnum, "Propane Modbus"=refnum}} {"Power"."Yokogawa"."WT310_3"."V Range (6: 600V)" items=["Auto", "15V", "30V", "60V", "150V", "300V", "600V"]; "Power"."Yokogawa"."WT310_3"."A Range (12: 20A)" items=["Auto", "5mA", "10mA", "20mA", "50mA", "100mA", "200mA", "0.5A", "1A", "2A", "5A", "10A", "20A", "50mV", "100mV", "200mV", "2.5V", "5V", "10V"]; "Power"."Yokogawa"."WT310_3"."Sample Rate (1: 0.25s)" items=["0.1s", "0.25s", "0.5s", "1s", "2s", "5s"]; "Power"."Yokogawa"."WT310_2"."V Range (6: 600V)" items=["Auto", "15V", "30V", "60V", "150V", "300V", "600V"]; "Power"."Yokogawa"."WT310_2"."A Range (12: 20A)" items=["Auto", "5mA", "10mA", "20mA", "50mA", "100mA", "200mA", "0.5A", "1A", "2A", "5A", "10A", "20A", "50mV", "100mV", "200mV", "2.5V", "5V", "10V"]; "Power"."Yokogawa"."WT310_2"."Sample Rate (1: 0.25s)" items=["0.1s", "0.25s", "0.5s", "1s", "2s", "5s"]; "Power"."Yokogawa"."WT500"."Update Rate (3: 500ms)" items=["-", "100ms", "200ms", "500ms", "1s", "2s", "5s"]; "Power"."Yokogawa"."WT500"."I Range (7: 40A)" items=["AUTO", "500 mA", "1 A", "2 A", "5 A", "10 A", "20 A", "40 A", "S-AUTO", "50 mV", "100 mV", "200 mV", "500 mV", "1 V", "2 V", "5 V", "10 V", "250 mA", "500 mA", "1 A", "2.5 A", "5 A", "10 A", "20 A", "25 mV", "50 mV", "100 mV", "250 mV", "500 mV", "1 V", "2.5 V", "5 V"]; "Power"."Yokogawa"."WT500"."V Range (8: 1000V)" items=["AUTO", "15", "30", "60", "100", "150", "300", "600", "1000", "7.5", "15", "30", "50", "75", "150", "300", "500"]; "Power"."Yokogawa"."WT210"."V Range (6: 600V)" items=["Auto", "15V", "30V", "60V", "150V", "300V", "600V"]; "Power"."Yokogawa"."WT210"."A Range (12: 20A)" items=["Auto", "5mA", "10mA", "20mA", "50mA", "100mA", "200mA", "0.5A", "1A", "2A", "5A", "10A", "20A", "50mV", "100mV", "200mV", "2.5V", "5V", "10V"]; "Power"."Yokogawa"."WT210"."Sample Rate (1: 0.25s)" items=["0.1s", "0.25s", "0.5s", "1s", "2s", "5s"]}, 16 "uA Output":i32, 19 "error out":errorcluster)   [LabVIEW 2023]
uses:
  Utility/Custom Pallet Controls/Custom Pallet DBL.ctl
  Type Definitions/HEWH Output Information.ctl
  Type Definitions/HEWH Draw Pattern Setup.ctl
  Type Definitions/PRAT Test.ctl
  Utility/Save File/File Setup (Public)/Type Definition/Save File HEWH Heating Control Mode.ctl
  Type Definitions/Terminate Draw Conditions.ctl
  Type Definitions/HEWH Start Conditions.ctl
  Type Definitions/Check Special Condtions.ctl
  Type Definitions/HEWH Special Condition Check.ctl
  Type Definitions/HEWH Draw Flag ENUM.ctl
  Type Definitions/HEWH Specific DAQ.ctl
  Type Definitions/HEWH Power Data.ctl
  Type Definitions/HEWH Power Elements.ctl
  Utility/Type Definitions/UTILITY Power Analyzer.ctl
  Type Definitions/HEWH Calc and Calibration.ctl
  Utility/Save File/File Setup (Public)/Type Definition/Save File DOE LabView Program.ctl
  Custom Instrument Control/MW100/Type Definitions/Station ID Selector.ctl
  Range/Type Definitions/RANGE ANSI Rate.ctl
  Custom Instrument Control/MW100/Type Definitions/HEWH Module 4 Relay Status.ctl
  Drivers/Inficon Fusion Micro GC/Type Definitions/Inficon Data.ctl
  Drivers/Alicat Gas Meter Driver/Sub-VIs/Data Cluster.ctl
  Washer DOE/Type Definitions/DOE Test Fixture Hardware.ctl
  <vilib>/NI/Modbus Library/API/Master/Modbus Master.lvclass
  Utility/Type Definitions/UTILITY Power Inputs Control.ctl
  Drivers/IND560 Scale Monitor/Type Definitions/IND560 Configuration.ctl
  Type Definitions/HEWH Agilent Cluster.ctl
  Utility/Type Definitions/UTILITY TC Coefficients.ctl
  Drivers/Omega FMA-1600A Series Gas Flow Meter/Type Definitions/FMA1600A COM Ports.ctl
  Drivers/Alicat Gas Meter Driver/Sub-VIs/Data Frame.ctl
  Drivers/Omega FMA-1600A Series Gas Flow Meter/Type Definitions/FMA1600A Units String.ctl
  Drivers/Alicat Gas Meter Driver/Sub-VIs/Units of Measure.ctl
  Drivers/Inficon Fusion Micro GC/Type Definitions/Inficon IP Address.ctl
  Custom Instrument Control/Intellifaucet/Type Definitions/INTELLIFAUCT Temp Flow.ctl
  Utility/Save File/File Setup.lvlib
panel:
  # "Totalizer Timer"
  # "Natural Gas"
  # "Propane"
  # "Draw Pattern Setup (24 Hour)"
  # "Totalizer Timer"
  # "Natural Gas"
  # "Propane"
  # "Draw Pattern Setup (24 Hour)"
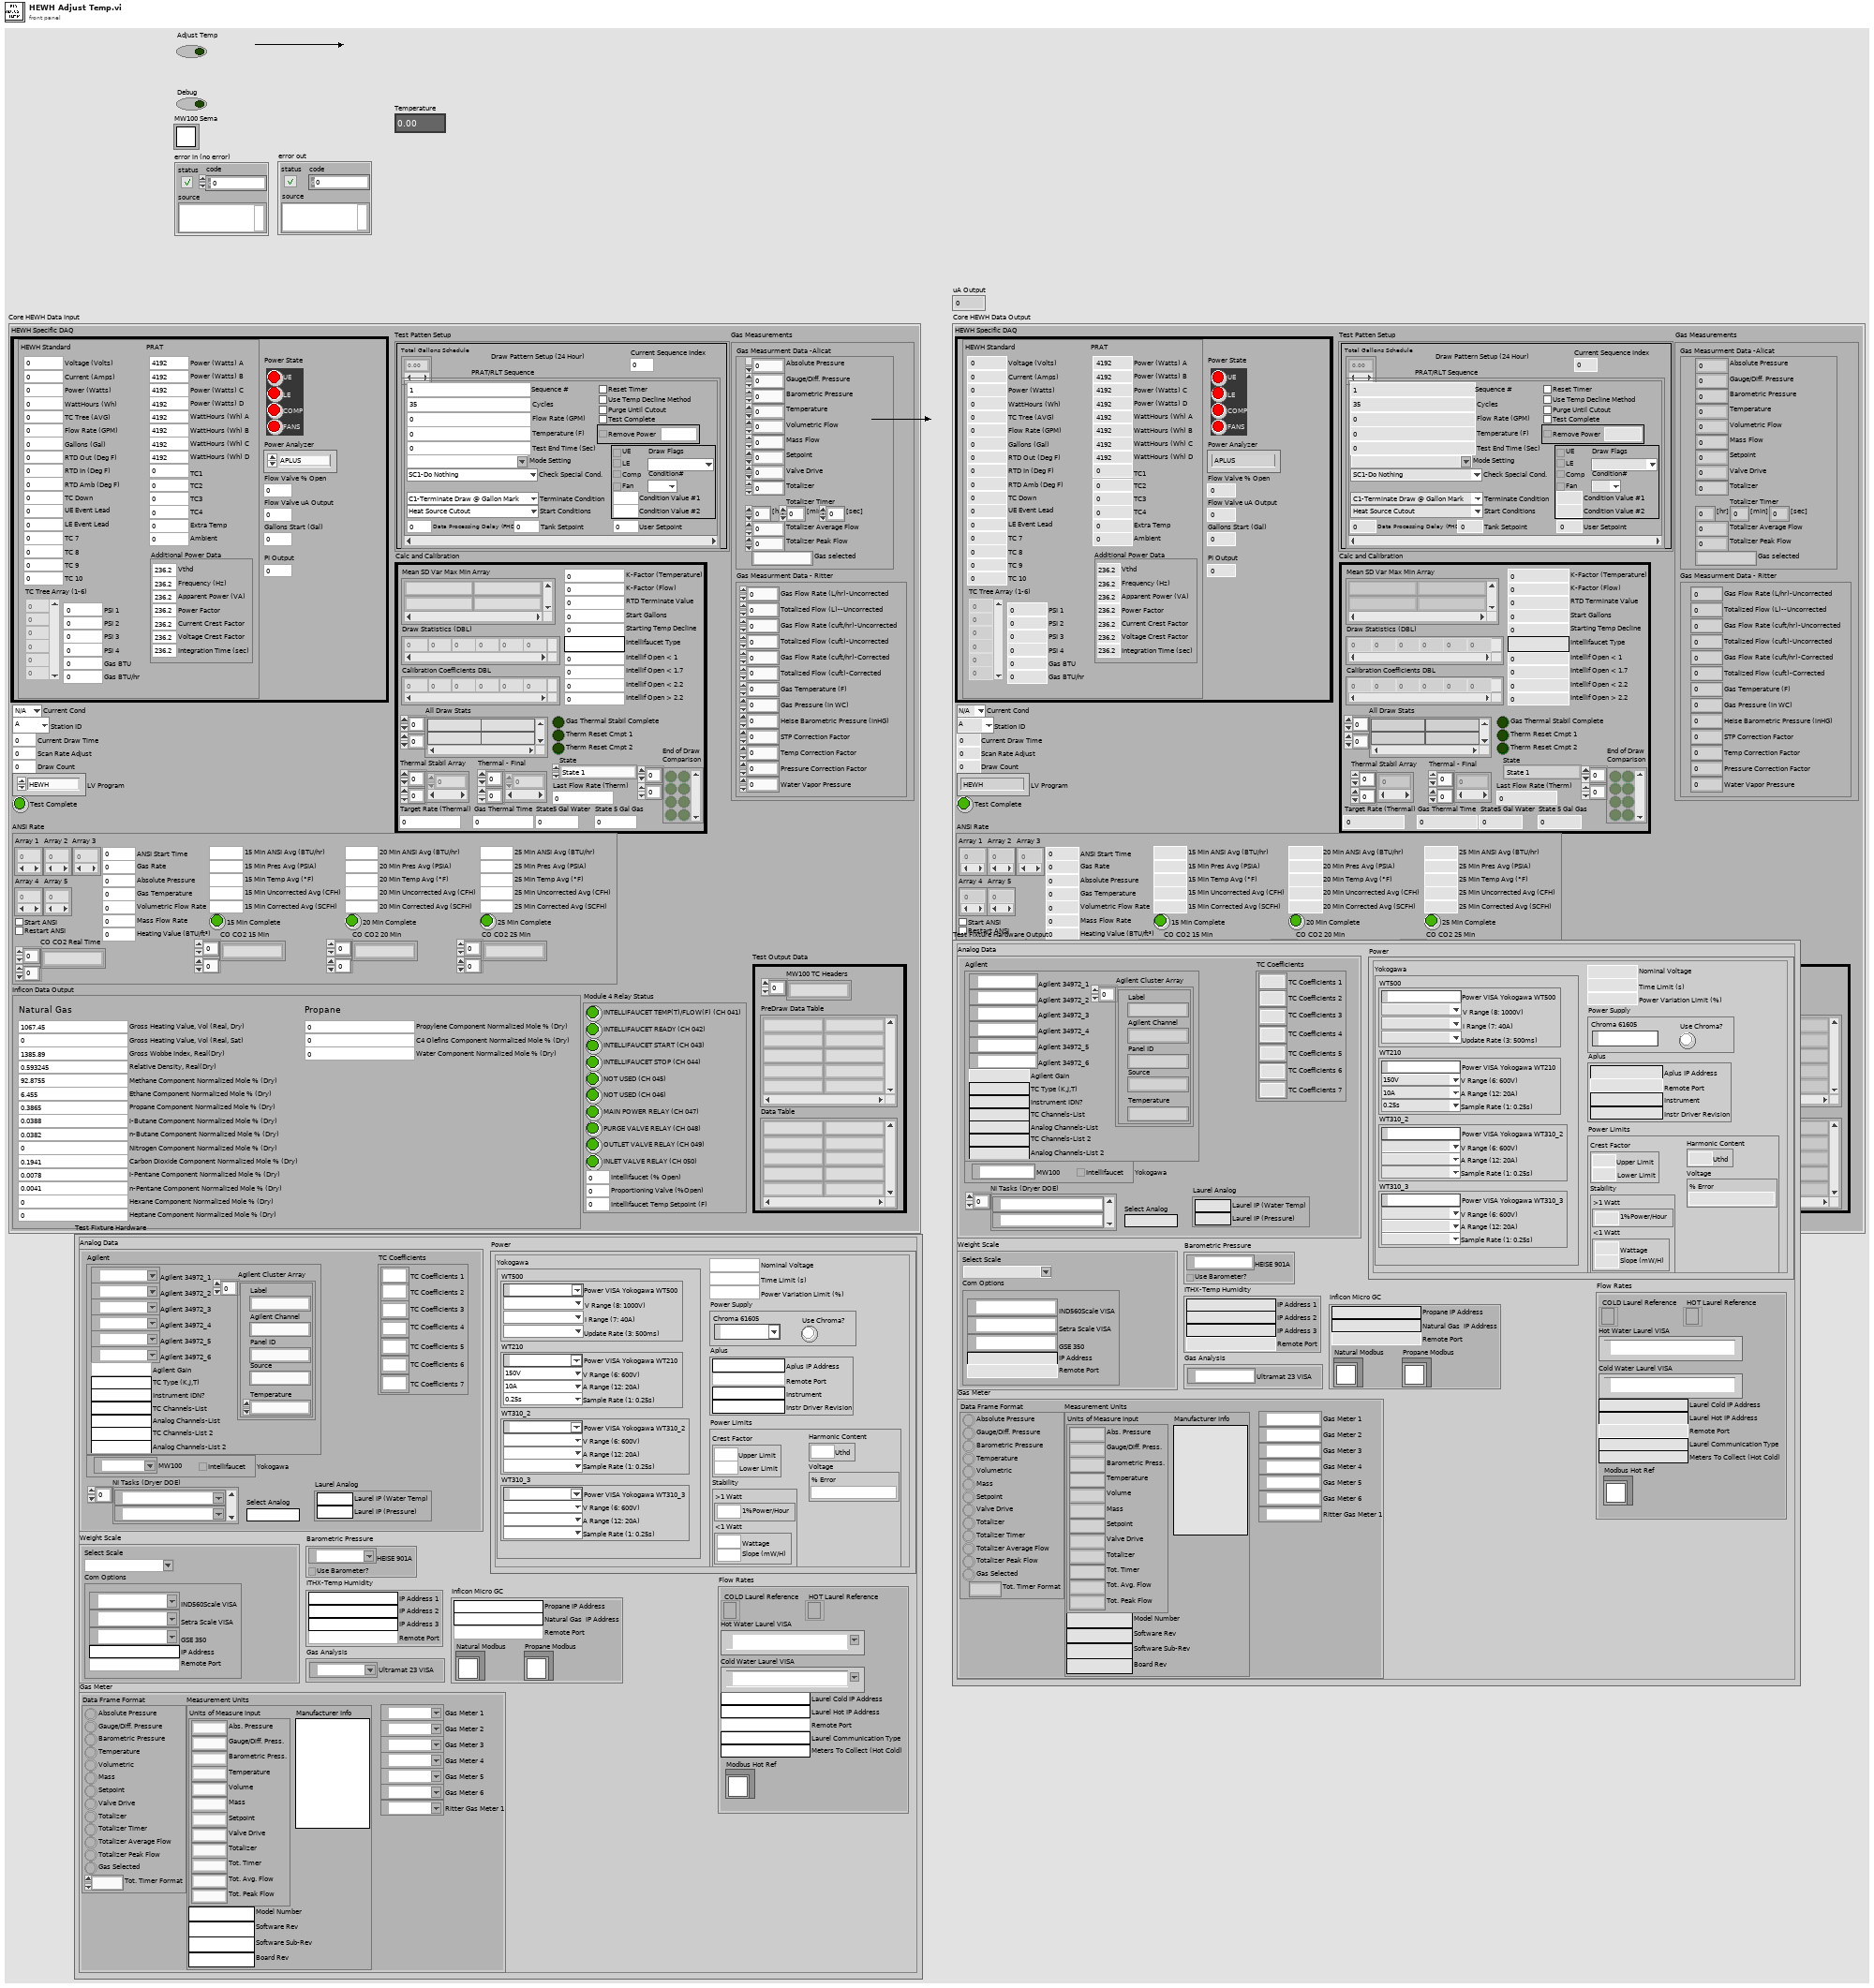
[diagram p1: front panel]
types:
  T1 = typedef "DOE Test Fixture Hardware.ctl" = cluster{"Power ":T2, "Weight Scale":cluster{"Com Options":T3, "Select Scale":string}, "Flow Rates":cluster{"Laurel Cold IP Address":string, "Laurel Hot IP Address":string, "Hot Water Laurel VISA":refnum<visa-resource-name>, "Cold Water Laurel VISA":refnum<visa-resource-name>, "Remote Port":u16, "Laurel Communication Type":string, "Meters To Collect (Hot Cold)":string, "HOT Laurel Reference":refnum<k5>, "COLD Laurel Reference":refnum<k5>, "Modbus Hot Ref":refnum<class "Modbus Master.lvclass">}, "Analog Data":cluster{"Agilent":cluster{"Agilent 34972_1":refnum<visa-resource-name>, "Agilent 34972_2":refnum<visa-resource-name>, "Agilent 34972_3":refnum<visa-resource-name>, "Agilent 34972_4":refnum<visa-resource-name>, "Agilent 34972_5":refnum<visa-resource-name>, "Agilent 34972_6":refnum<visa-resource-name>, "Agilent Gain":dbl, "TC Type (K,J,T)":string, "Instrument IDN?":string, "TC Channels-List":string, "Analog Channels-List":string, "Agilent Cluster Array":T4[], "TC Channels-List 2":string, "Analog Channels-List 2":string}, "Yokogawa":cluster{"MW100":refnum<visa-resource-name>, "Intellifaucet":bool}, "Select Analog":string, "TC Coefficients":T5, "NI Tasks (Dryer DOE)":refnum<k21>[], "Laurel Analog":cluster{"Laurel IP (Water Temp)":string, "Laurel IP (Pressure)":string}}, "ITHX-Temp Humidity":cluster{"IP Address 1":string, "Remote Port":u16, "IP Address 2":string, "IP Address 3":string}, "Gas Meter":T6, "Barometric Pressure":cluster{"HEISE 901A":refnum<visa-resource-name>, "Use Barometer?":bool}, "Gas Analysis":cluster{"Ultramat 23 VISA":refnum<visa-resource-name>}, "Inficon Micro GC":T10}
  T2 = typedef "UTILITY Power Inputs Control.ctl" = cluster{"Yokogawa":cluster{"WT210":cluster{"Sample Rate (1: 0.25s)":i32, "A Range (12: 20A)":i32, "V Range (6: 600V)":i32, "Power VISA Yokogawa WT210":refnum<visa-resource-name>}, "WT500":cluster{"Power VISA Yokogawa WT500":refnum<visa-resource-name>, "V Range (8: 1000V)":i32, "I Range (7: 40A)":i32, "Update Rate (3: 500ms)":i32}, "WT310_2":cluster{"Sample Rate (1: 0.25s)":i32, "A Range (12: 20A)":i32, "V Range (6: 600V)":i32, "Power VISA Yokogawa WT310_2":refnum<visa-resource-name>}, "WT310_3":cluster{"Sample Rate (1: 0.25s)":i32, "A Range (12: 20A)":i32, "V Range (6: 600V)":i32, "Power VISA Yokogawa WT310_3":refnum<visa-resource-name>}}, "Aplus":cluster{"Aplus IP Address":string, "Remote Port":i32, "Instrument":string, "Instr Driver Revision":string}, "Power Limits":cluster{"Crest Factor":cluster{"Upper Limit":dbl, "Lower Limit":dbl}, "Harmonic Content":cluster{"Uthd":dbl}, "Voltage":cluster{"% Error":dbl}, "Stability":cluster{"<1 Watt ":cluster{"Wattage":dbl, "Slope (mW/H)":dbl}, ">1 Watt":cluster{"1%Power/Hour":dbl}}}, "Nominal Voltage":i32, "Time Limit (s)":dbl, "Power Variation Limit (%)":dbl, "Power Supply":cluster{"Chroma 61605":refnum<visa-resource-name>, "Use Chroma?":bool}}
  T3 = typedef "IND560 Configuration.ctl" = cluster{"IND560Scale VISA":refnum<visa-resource-name>, "IP Address":string, "Remote Port":u16, "Setra Scale VISA":refnum<visa-resource-name>, "GSE 350":refnum<visa-resource-name>}
  T4 = typedef "HEWH Agilent Cluster.ctl" = cluster{"Label":string, "Agilent Channel":string, "Panel ID":string, "Source":string, "Temperature":dbl}
  T5 = typedef "UTILITY TC Coefficients.ctl" = cluster{"TC Coefficients 1":dbl[], "TC Coefficients 2":dbl[], "TC Coefficients 3":dbl[], "TC Coefficients 4":dbl[], "TC Coefficients 5":dbl[], "TC Coefficients 6":dbl[], "TC Coefficients 7":dbl[]}
  T6 = typedef "FMA1600A COM Ports.ctl" = cluster{"Gas Meter 1":refnum<visa-resource-name>, "Gas Meter 2":refnum<visa-resource-name>, "Gas Meter 3":refnum<visa-resource-name>, "Gas Meter 4":refnum<visa-resource-name>, "Gas Meter 5":refnum<visa-resource-name>, "Gas Meter 6":refnum<visa-resource-name>, "Data Frame Format":T7, "Measurement Units":T8, "Ritter Gas Meter 1":refnum<visa-resource-name>}
  T7 = typedef "Data Frame.ctl" = cluster{"Absolute Pressure":bool, "Gauge/Diff. Pressure":bool, "Barometric Pressure":bool, "Temperature":bool, "Volumetric":bool, "Mass":bool, "Setpoint":bool, "Valve Drive":bool, "Totalizer":bool, "Totalizer Timer":bool, "Totalizer Average Flow":bool, "Totalizer Peak Flow":bool, "Gas Selected":bool, "Tot. Timer Format":u16}
  T8 = typedef "FMA1600A Units String.ctl" = cluster{"Software Rev":string, "Model Number":string, "Manufacturer Info":string, "Software Sub-Rev":string, "Board Rev":string, "Units of Measure Input":T9}
  T9 = typedef "Units of Measure.ctl" = cluster{"Abs. Pressure":string, "Gauge/Diff. Press.":string, "Barometric Press.":string, "Temperature":string, "Volume":string, "Mass":string, "Setpoint":string, "Valve Drive":string, "Totalizer":string, "Tot. Timer":string, "Tot. Avg. Flow":string, "Tot. Peak Flow":string}
  T10 = typedef "Inficon IP Address.ctl" = cluster{"Propane IP Address":string, "Natural Gas  IP Address":string, "Remote Port":u16, "Natural Modbus":refnum<class "Modbus Master.lvclass">, "Propane Modbus":refnum<class "Modbus Master.lvclass">}
  T11 = typedef "Semaphore RefNum" = refnum<k1>
  T12 = typedef "HEWH Output Information.ctl" = cluster{"Scan Rate Adjust":dbl, "Draw Count":i32, "Test Patten Setup":T13, "HEWH Specific DAQ":T21, "Test Output Data":cluster{"PreDraw Data Table":string[][], "Data Table":string[][], "MW100 TC Headers":string[]}, "Calc and Calibration":T25, "Current Draw Time":dbl, "LV Program":T26, "Station ID":T27, "Current Cond":T19, "Test Complete":bool, "ANSI Rate":T28, "Module 4 Relay Status":T29, "Inficon Data Output":T30, "Gas Measurements":cluster{"Gas Measurment Data -Alicat":T31, "Gas Measurment Data - Ritter":cluster{"Gas Flow Rate (L/hr)-Uncorrected":dbl, "Totalized Flow (L)--Uncorrected":dbl, "Gas Flow Rate (cuft/hr)-Uncorrected":dbl, "Totalized Flow (cuft)-Uncorrected":dbl, "Gas Temperature (F)":dbl, "Gas Pressure (in WC)":dbl, "Heise Barometric Pressure (inHG)":dbl, "STP Correction Factor":dbl, "Temp Correction Factor":dbl, "Pressure Correction Factor":dbl, "Water Vapor Pressure":dbl, "Gas Flow Rate (cuft/hr)-Corrected":dbl, "Totalized Flow (cuft)-Corrected":dbl}}}
  T13 = typedef "HEWH Draw Pattern Setup.ctl" = cluster{"Total Gallons Schedule":dbl[], "PRAT/RLT Sequence":T14[], "Current Sequence Index":i32}
  T14 = typedef "PRAT Test.ctl" = cluster{"Sequence #":dbl, "Cycles":i32, "Mode Setting":T15, "Flow Rate (GPM)":dbl, "Temperature (F)":dbl, "Reset Timer":bool, "Use Temp Decline Method":bool, "Terminate Condition":T16, "Condition Value #1":dbl, "UE":bool, "LE":bool, "Comp":bool, "Fan":bool, "Test End Time (Sec)":dbl, "Purge Until Cutout":bool, "Start Conditions":T17, "Condition Value #2":dbl, "Remove Power":bool, "Time":dbl, "Check Special Cond.":T18, "Condition#":T19, "Draw Flags":T20, "Data Processing Delay (FHD 15sec, UEF 5 Sec)":dbl, "Test Complete":bool, "User Setpoint":dbl, "Tank Setpoint":dbl}
  T15 = typedef "File Setup.lvlib/Save File HEWH Heating Control Mode.ctl" = string
  T16 = typedef "Terminate Draw Conditions.ctl" = enum16{"C1-Terminate Draw @ Gallon Mark", "C2-Special Last Draw (HU Test)", "C3-RTD Out <=", "C4-Mean Tank Temp <=", "C5-Decrease RTD Out (Deg F)", "C6-Time (Seconds)", "C7-Until Any Heat Source", "C8-Specific Heat Source", "C9-Do Nothing", "C10-Inlet Outlet RTD Temp Delta"}
  T17 = typedef "HEWH Start Conditions.ctl" = enum16{"Heat Source Cutout", "At Time (Seconds)", "Every X (Seconds)", "T2 >= X° Below Setpoint", "Seconds From Complete", "Wait for LE & Comp Cutout", "Wait for Comp Cutout", "Wait for LE Cutout", "Wait for UE Cutout", "Start Immediately"}
  T18 = typedef "Check Special Condtions.ctl" = enum16{"SC1-Do Nothing", "SC2-Check Heat Source (On-C2/Off-C1)", "SC3-Check Skip Condition", "SC4-Check Heat Source ON/Fail", "SC5-Keep Draw Valves Open", "SC6-Skip Purge"}
  T19 = typedef "HEWH Special Condition Check.ctl" = enum16{"N/A", "C1", "C2", "Reset/Fail", "Skip Draw Sequence"}
  T20 = typedef "HEWH Draw Flag ENUM.ctl" = enum16{"N/A", "None(0)", "Sml(1)", "Med(2)", "SmlMed(3)", "Lrg(4)", "SmlLrg(5)", "MedLrg(6)", "SmlMedLrg(7)"}
  T21 = typedef "HEWH Specific DAQ.ctl" = cluster{"HEWH Data":T22, "Flow Valve % Open":dbl, "Power State":T23, "Power Analyzer":T24, "Flow Valve uA Output":i32, "Gallons Start (Gal)":dbl, "PI Output":dbl}
  T22 = typedef "HEWH Power Data.ctl" = cluster{"HEWH Standard":cluster{"Voltage (Volts)":dbl, "Current (Amps)":dbl, "Power (Watts)":dbl, "WattHours (Wh)":dbl, "TC Tree (AVG)":dbl, "Flow Rate (GPM)":dbl, "Gallons (Gal)":dbl, "RTD Out (Deg F)":dbl, "RTD In (Deg F)":dbl, "RTD Amb (Deg F)":dbl, "TC Down":dbl, "UE Event Lead":i32, "LE Event Lead":i32, "TC 8":dbl, "TC 9":dbl, "TC 10":dbl, "TC Tree Array (1-6)":dbl[], "TC 7":dbl, "PSI 1":dbl, "PSI 2":dbl, "PSI 3":dbl, "PSI 4":dbl, "Gas BTU":dbl, "Gas BTU/hr":dbl}, "PRAT":cluster{"Power (Watts) A":dbl, "Power (Watts) B":dbl, "Power (Watts) C":dbl, "Power (Watts) D":dbl, "TC1":dbl, "TC2":dbl, "TC3":dbl, "TC4":dbl, "WattHours (Wh) A":dbl, "WattHours (Wh) B":dbl, "WattHours (Wh) C":dbl, "WattHours (Wh) D":dbl, "Ambient":dbl, "Extra Temp":dbl}, "Additional Power Data":cluster{"Vthd":dbl, "Frequency (Hz)":dbl, "Apparent Power (VA)":dbl, "Power Factor":dbl, "Current Crest Factor":dbl, "Voltage Crest Factor":dbl, "Integration Time (sec)":dbl}}
  T23 = typedef "HEWH Power Elements.ctl" = cluster{"UE":bool, "LE":bool, "COMP":bool, "FANS":bool}
  T24 = typedef "UTILITY Power Analyzer.ctl" = enum16{"", "APLUS", "WT210", "WT500", "WT300", "OSI", "Debug", "WT230", "WT300_1", "WT300_2"}
  T25 = typedef "HEWH Calc and Calibration.ctl" = cluster{"Mean SD Var Max Min Array":string[][], "Draw Statistics (DBL)":dbl[][], "Calibration Coefficients DBL":dbl[][], "Start Gallons":dbl, "Starting Temp Decline":dbl, "K-Factor (Temperature)":dbl, "All Draw Stats":string[][], "RTD Terminate Value":dbl, "K-Factor (Flow)":dbl, "Intellifaucet Type":string, "Thermal Stabil Array":dbl[][], "Gas Thermal Stabil Complete":bool, "Therm Reset Cmpt 1":bool, "Therm Reset Cmpt 2":bool, "Last Flow Rate (Therm)":dbl, "State":enum16{"State 0", "State 1", "State 2", "State 3", "State 4", "State 5", "State 6"}, "Gas Thermal Time":dbl, "Target Rate (Thermal)":dbl, "Thermal - Final":dbl[][], "State5 Gal Water":dbl, "State 5 Gal Gas":dbl, "Intellif Open < 1":dbl, "Intellif Open < 1.7":dbl, "Intellif Open < 2.2":dbl, "Intellif Open > 2.2":dbl, "End of Draw\nComparison":bool[][]}
  T26 = typedef "File Setup.lvlib/Save File DOE LabView Program.ctl" = enum16{"No Name Found", "DOE Stand", "Dishwasher Kitchen", "Portable Stand", "HEWH", "Dryer", "Dryer WILT", "HCC", "PRAT", "HEWH RLT", "Refrigeration", "Gas Water Heater"}
  T27 = typedef "Station ID Selector.ctl" = enum16{"", "A", "B", "C", "D", "Global"}
  T28 = typedef "RANGE ANSI Rate.ctl" = cluster{"Array 1":dbl[], "Array 3":dbl[], "Array 2":dbl[], "Start ANSI":bool, "ANSI Start Time":dbl, "Restart ANSI":bool, "15 Min ANSI Avg (BTU/hr)":dbl, "20 Min ANSI Avg (BTU/hr)":dbl, "25 Min ANSI Avg (BTU/hr)":dbl, "Absolute Pressure":dbl, "Gas Temperature":dbl, "Volumetric Flow Rate":dbl, "Mass Flow Rate":dbl, "Array 4":dbl[], "Array 5":dbl[], "Gas Rate":dbl, "15 Min Pres Avg (PSIA)":dbl, "20 Min Pres Avg (PSIA)":dbl, "25 Min Pres Avg (PSIA)":dbl, "15 Min Temp Avg (°F) ":dbl, "20 Min Temp Avg (°F)":dbl, "25 Min Temp Avg (°F)":dbl, "15 Min Uncorrected Avg (CFH)":dbl, "20 Min Uncorrected Avg (CFH)":dbl, "25 Min Uncorrected Avg (CFH)":dbl, "15 Min Corrected Avg (SCFH)":dbl, "20 Min Corrected Avg (SCFH)":dbl, "25 Min Corrected Avg (SCFH)":dbl, "15 Min Complete":bool, "20 Min Complete":bool, "25 Min Complete":bool, "Heating Value (BTU/ft³)":dbl, "CO CO2 15 Min":string[][], "CO CO2 20 Min":string[][], "CO CO2 25 Min":string[][], "CO CO2 Real Time":string[][]}
  T29 = typedef "HEWH Module 4 Relay Status.ctl" = cluster{"INTELLIFAUCET TEMP(T)/FLOW(F) (CH 041)":bool, "INTELLIFAUCET READY (CH 042)":bool, "INTELLIFAUCET START (CH 043)":bool, "INTELLIFAUCET STOP (CH 044)":bool, "MAIN POWER RELAY (CH 047)":bool, "NOT USED (CH 045)":bool, "NOT USED (CH 046)":bool, "PURGE VALVE RELAY (CH 048)":bool, "OUTLET VALVE RELAY (CH 049)":bool, "INLET VALVE RELAY (CH 050)":bool, "Intellifaucet (% Open)":dbl, "Proportioning Valve (%Open)":dbl, "Intellifaucet Temp Setpoint (F)":dbl}
  T30 = typedef "Inficon Data.ctl" = cluster{"Gross Heating Value, Vol (Real, Dry)":dbl, "Nitrogen Component Normalized Mole % (Dry)":dbl, "Methane Component Normalized Mole % (Dry)":dbl, "Carbon Dioxide Component Normalized Mole % (Dry)":dbl, "Ethane Component Normalized Mole % (Dry)":dbl, "Propane Component Normalized Mole % (Dry)":dbl, "i-Pentane Component Normalized Mole % (Dry)":dbl, "i-Butane Component Normalized Mole % (Dry)":dbl, "n-Butane Component Normalized Mole % (Dry)":dbl, "n-Pentane Component Normalized Mole % (Dry)":dbl, "Hexane Component Normalized Mole % (Dry)":dbl, "Heptane Component Normalized Mole % (Dry)":dbl, "Gross Wobbe Index, Real(Dry)":dbl, "Relative Density, Real(Dry)":dbl, "Propylene Component Normalized Mole % (Dry)":dbl, "C4 Olefins Component Normalized Mole % (Dry)":dbl, "Water Component Normalized Mole % (Dry)":dbl, "Gross Heating Value, Vol (Real, Sat)":dbl}
  T31 = typedef "Data Cluster.ctl" = cluster{"Absolute Pressure":dbl, "Gauge/Diff. Pressure":dbl, "Barometric Pressure":dbl, "Temperature":dbl, "Volumetric Flow":dbl, "Mass Flow":dbl, "Setpoint":dbl, "Valve Drive":dbl, "Totalizer":dbl, "[hr]":dbl, "[min]":dbl, "[sec]":dbl, "Totalizer Average Flow":dbl, "Totalizer Peak Flow":dbl, "Gas selected":string}
  T32 = typedef "Custom Pallet DBL.ctl" = dbl
  T33 = typedef "INTELLIFAUCT Temp Flow.ctl" = enum8{"TEMP", "FLOW", "Prop Valve"}
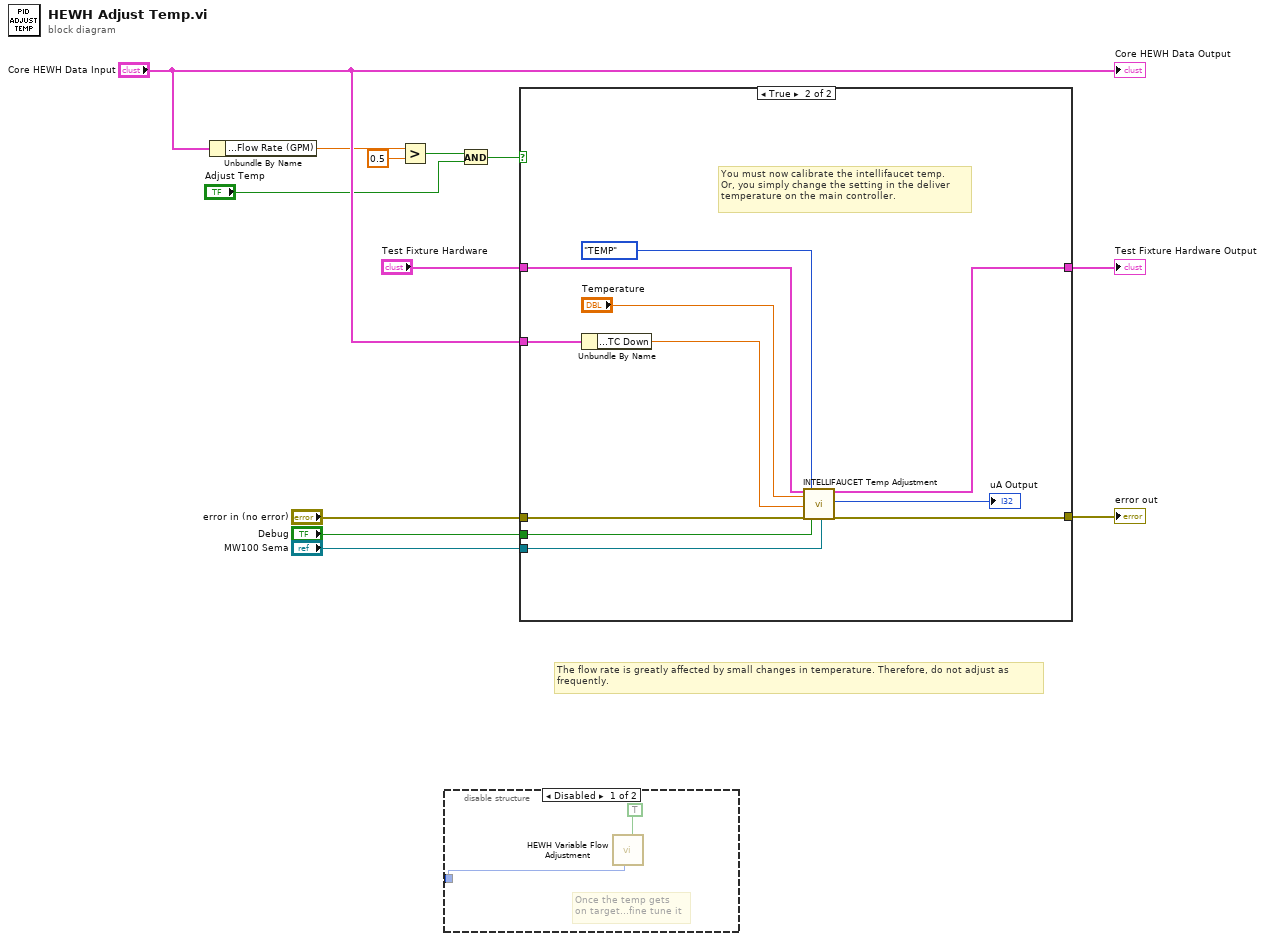
[diagram p0: block diagram]
diagram:
  # "The flow rate is greatly affected by small changes in temperature. Therefore, do not adjust as\nfrequently."
  n1 = Unbundle By Name("Core HEWH Data Input") -> ("HEWH Specific DAQ.HEWH Data.HEWH Standard.Flow Rate (GPM)"=w5:dbl)
  n2 = Greater?(x=w5, y=0.5) -> (0:w3:bool)
  n3 = disable-structure shown="Disabled" {
    disable-tunnel: _ -> [w13 _]
    frame Disabled {
      # "Once the temp gets \non target...fine tune it"
      n4 = call "HEWH Variable Flow Adjustment.vi"("Temp (T) or Flow (F)"=TRUE, "State in"=w13) -> ()  [unwired: 9 in, 1 out]
    }
    frame Enabled {
    }
  }
  n5 = And(x=w3, y="Adjust Temp") -> (x .and. y?=w1:bool)
  n6 = case shown="True" w1 {
    tunnel: "Test Fixture Hardware" -> [w16 w27]
    tunnel: "Core HEWH Data Input" -> [_ w20]
    tunnel: "error in (no error)" -> [w15 w26]
    tunnel: "Debug" -> [_ w25]
    tunnel: "MW100 Sema" -> [_ w24]
    tunnel: [w15 w23] -> w12
    tunnel: [w16 w22] -> w8
    frame False {
    }
    frame True {
      # "You must now calibrate the intellifaucet temp. \nOr, you simply change the setting in the deliver\ntemperature on the main controller."
      n7 = Unbundle By Name(w20) -> ("HEWH Specific DAQ.HEWH Data.HEWH Standard.TC Down"=w17:dbl)
      n8 = call "INTELLIFAUCET Temp Adjustment.vi"("Test Fixture Hardware"=w27, "Target"="Temperature", "Reading"=w17, "Error In"=w26, "TEMP,FLOW"=INTELLIFAUCT_Temp_Flow."TEMP", "Debug"=w25, "Refnum in"=w24) -> ("Test Fixture Hardware Output"=w22:T1, "uA Output"=→"uA Output":i32, "Error Out"=w23:errorcluster)  [unwired: 9 in, 1 out]
    }
  }
  "error out" <- w12
  "Test Fixture Hardware Output" <- w8
  "Core HEWH Data Output" <- "Core HEWH Data Input"
